vi "roboRIO v1.0 Reserve I2C.vi"(7 "Allow multiple opens?":bool, 8 "error in (no error)":errorcluster, 10 "I2C Channel":T2, 11 "myRIO FPGA Ref Out":T1) -> (0 "error out":errorcluster)   [LabVIEW 2021]
uses:
  <vilib>/myRIO/Common/Instrument Driver Framework/myRIO v1.0/I2C/typedefs/I2C Channels Enum.ctl
  <vilib>/myRIO/Common/Instrument Driver Framework/Utilities/typedefs/Generic FPGA Reference.ctl
  <vilib>/myRIO/Common/Instrument Driver Framework/roboRIO v1.0/Resource Manager/vis/roboRIO v1.0 Reserve Channel.vi
  <vilib>/myRIO/Common/Instrument Driver Framework/roboRIO v1.0/Resource Manager/vis/roboRIO v1.0 Unreserve Channel.vi
  <vilib>/myRIO/Common/Instrument Driver Framework/roboRIO v1.0/Resource Manager/vis/roboRIO v1.0 Create Configuration List.vi
  <vilib>/myRIO/Common/Instrument Driver Framework/roboRIO v1.0/Resource Manager/vis/roboRIO v1.0 Build Mutex Name.vi
  <vilib>/myRIO/Common/Instrument Driver Framework/Utilities/vis/IO Manager.vi
  <vilib>/Utility/error.llb/Error Cluster From Error Code.vi
  <vilib>/myRIO/Common/Instrument Driver Framework/Utilities/vis/Configuration Manager.vi
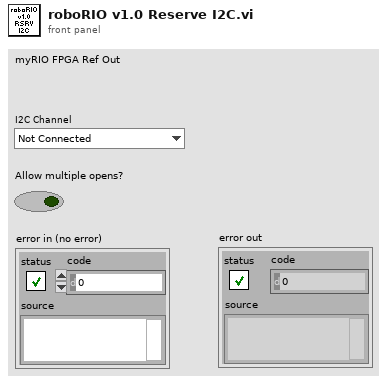
[diagram p1: front panel]
types:
  T1 = typedef "Generic FPGA Reference.ctl" = refnum<k20>
  T2 = typedef "I2C Channels Enum.ctl" = enum16{"Not Connected", "A/I2C", "B/I2C", "I2C/I2C"}
  T3 = typedef "roboRIO v1.0 Channel Reservation List.ctl" = T4[]
  T4 = typedef "roboRIO v1.0 Channel Reservation Info.ctl" = cluster{"Channel Name":string, "Connector":T5, "Mutex ID":i32}
  T5 = typedef "roboRIO v1.0 Connector List.ctl" = enum32{"None", "ConnectorB", "ConnectorI2C", "ConnectorDIO", "ConnectorRSL", "ConnectorRELAY", "ConnectorAI", "ConnectorPWM", "ConnectorSPI"}
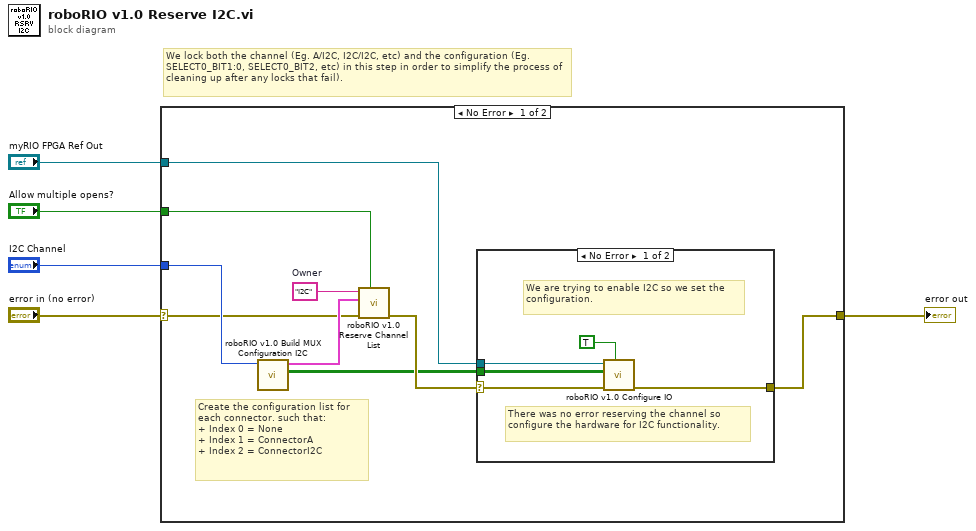
[diagram p0: block diagram]
diagram:
  # "We lock both the channel (Eg. A/I2C, I2C/I2C, etc) and the configuration (Eg. SELECT0_BIT1:0, SELECT0_BIT2, etc) in this step in order to simplify the process of cleaning up after any locks that fail)."
  n1 = case shown="No Error" "error in (no error)" {
    selector: "error in (no error)" -> [w7 w21]
    tunnel: "myRIO FPGA Ref Out" -> [w11 _]
    tunnel: "I2C Channel" -> [w14 _]
    tunnel: [w10 w21] -> w3
    tunnel: "Allow multiple opens?" -> [w13 _]
    frame No Error {
      w12 = "I2C"  # Owner
      # "Create the configuration list for each connector. such that:\n+ Index 0 = None\n+ Index 1 = ConnectorA\n+ Index 2 = ConnectorI2C"
      n2 = call <vilib>:"roboRIO v1.0 Build MUX Configuration I2C.vi"("Channel"=w14) -> ("Configuration Bitmask Array"=w6:bool[][], "Channel Reservation List"=w9:T3)  [unwired: 9 in]
      n3 = call <vilib>:"roboRIO v1.0 Reserve Channel List.vi"("Allow multiple opens?"=w13, "error in (no error)"=w7, "Channel Reservation List"=w9, "Owner"=w12) -> ("error out"=w8:errorcluster)  [unwired: 7 in]
      n4 = case shown="No Error" w8 {
        selector: w8 -> [w16 w20]
        tunnel: w11 -> [w18 _]
        tunnel: [w17 w20] -> w10
        tunnel: w6 -> [w15 _]
        frame No Error {
          # "We are trying to enable I2C so we set the configuration."
          # "There was no error reserving the channel so configure the hardware for I2C functionality."
          n5 = call <vilib>:"roboRIO v1.0 Configure IO.vi"("Value"=TRUE ("Clear?"), "error in (no error)"=w16, "Bitmask Array"=w15, "myRIO FPGA Ref In"=w18) -> ("error out"=w17:errorcluster)  [unwired: 7 in]
        }
        frame Error {
        }
      }
    }
    frame Error {
      # "Nothing to do since there is an incoming error."
    }
  }
  "error out" <- w3
